vi "DemoSubClass2_SetModifiedAttributes.vi"(0 "reference in":refnum<class "DemoSubClass2.lvclass">, 2 "Attributes":T1 {"Base class"."Attribute1" format="%.2f"}, 3 "Only unlock data? (F)":bool, 4 "Unlock data if error? (T)":bool=TRUE, 5 "error in (no error)":errorcluster, 7 "Update data even if error? (F)":bool) -> (14 "reference out":refnum<class "DemoSubClass2.lvclass">, 19 "error out":errorcluster)   [LabVIEW 2020, in "DemoSubClass2.lvclass"]
doc: "This VI overwrites the attributes associated with the object reference and unlocks it for write access. If error in is set, the object is unlocked but its data will not be modified.\n\nIn order to use this VI, you must first successfully lock the object's data using this class GetAttributesToModify VI."
uses:
  DemoSubClass2.lvclass
  protected/ObjectAttributes.ctl
  DemoClass1_class/protected/ObjectAttributes.ctl
  DemoSubClass2.lvclass/DemoSubClass2.ctl
  _goop3.llb/3GOOPStates.ctl
  DemoClass1_class/DemoClass1.lvclass
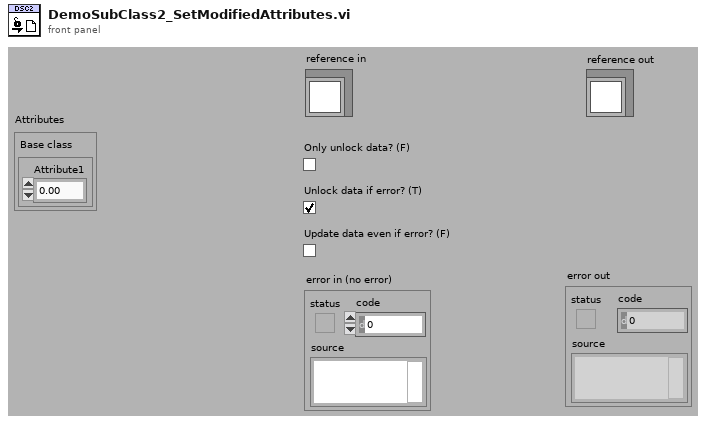
[diagram p1: front panel]
types:
  T1 = typedef "DemoSubClass2.lvclass/ObjectAttributes.ctl" = cluster{"Base class":T2}
  T2 = typedef "DemoClass1.lvclass/ObjectAttributes.ctl" = cluster{"Attribute1":dbl}
  T3 = typedef "DemoClass1.lvclass/ObjectReference.ctl" = refnum<k1>
  T4 = typedef "3GOOPStates.ctl" = enum16{"Set", "Get", "New", "Delete", "Clear", "Test and get", "Unlock data", "Information", "Look up existing", "New or look up existing", "Test and get shared", "Get shared", "Set shared", "Unlock shared", "Find dynamic method", "Register dynamic method", "Preload dynamic method", "Probe", "Cast to more generic", "Cast to more specific"}
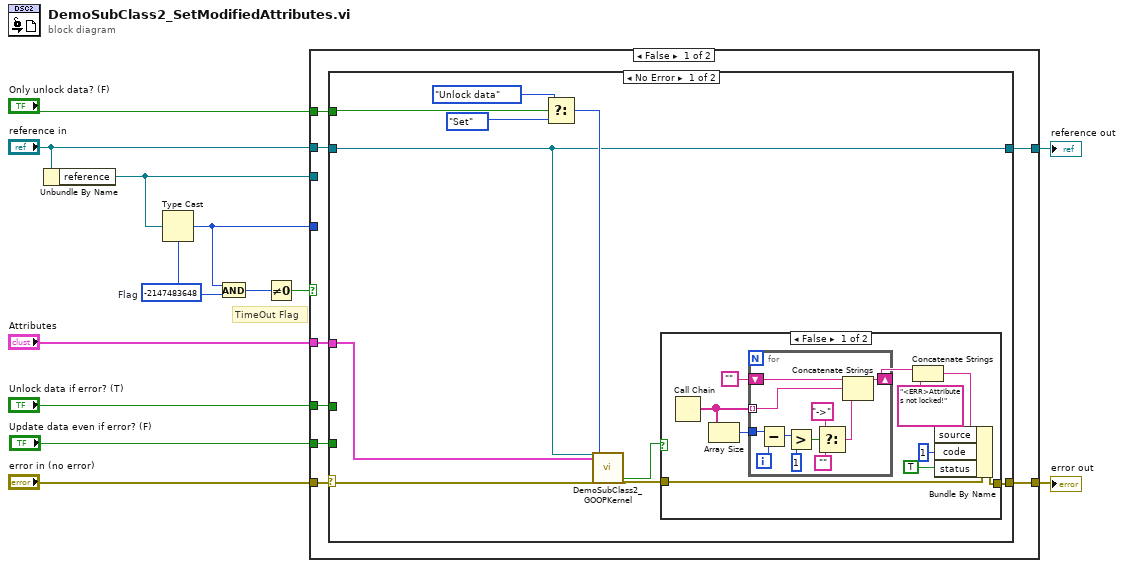
[diagram p0: block diagram]
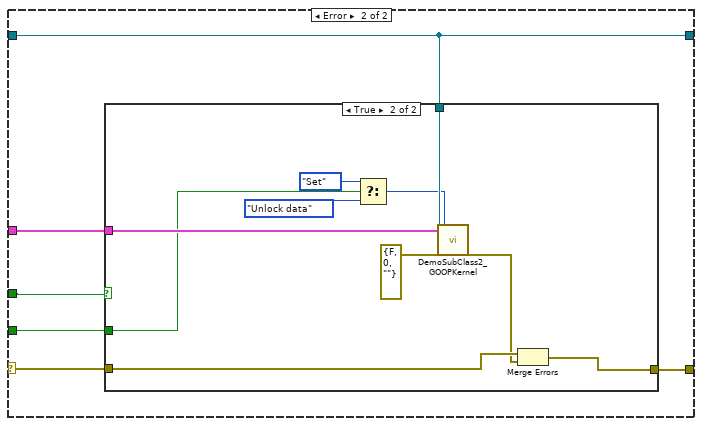
[diagram p3: hidden frame]
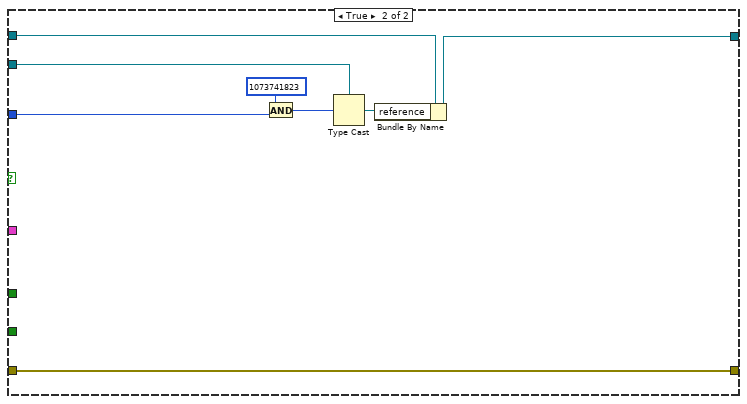
[diagram p5: hidden frame]
diagram:
  w2 = -2147483648  # Flag
  # "TimeOut Flag"
  n1 = Unbundle By Name("reference in") -> ("reference"=w5:T3)
  n2 = Type Cast(type=w2, x=w5) -> (*(type *) &x=w3:i32)
  n3 = And(x=w3, y=w2) -> (x .and. y?=w7:i32)
  n4 = Not Equal To 0?(x=w7) -> (x != 0?=w6:bool)
  n5 = case shown="False" w6 {
    tunnel: "Unlock data if error? (T)" -> [w21 _]
    tunnel: "error in (no error)" -> [w20 w71]
    tunnel: "Attributes" -> [w19 _]
    tunnel: "Only unlock data? (F)" -> [w18 _]
    tunnel: [w17 w74] -> w9
    tunnel: [w16 w71] -> w8
    tunnel: "reference in" -> [w15 w75]
    tunnel: w5 -> [_ w73]
    tunnel: w3 -> [_ w72]
    tunnel: "Update data even if error? (F)" -> [w14 _]
    frame False {
      n6 = case shown="No Error" w20 {
        selector: w20 -> [w30 w57]
        tunnel: [w22 w55] -> w17
        tunnel: w19 -> [w26 w59]
        tunnel: [w25 w56] -> w16
        tunnel: w15 -> [w22 w55]
        tunnel: w18 -> [w31 _]
        tunnel: w21 -> [_ w58]
        tunnel: w14 -> [_ w54]
        frame No Error {
          n7 = Select(t=3GOOPStates."Unlock data" ("Action"), s=w31, f=3GOOPStates."Set" ("Action")) -> (s? t:f=w27:T4)
          n8 = call "DemoSubClass2_GOOPKernel.vi"("Ref in"=w22, "Data in"=w26, "error in (no error)"=w30, "Action"=w27) -> ("Data locked?"=w23:bool, "error out"=w24:errorcluster)  [unwired: 13 in, 9 out]
          n9 = case shown="False" w23 {
            tunnel: w24 -> [w36 w53]
            tunnel: [w37 w53] -> w25
            frame False {
              n10 = Call Chain() -> (call chain=w32:string[])
              n11 = Array Size(array=w32) -> (size(s)=w40:i32)
              n12 = for {
                shift-right: [w46] -> w39
                shift-left: "" -> [w48]
                tunnel: w32 -> [w47] mode=indexing
                tunnel: w40 -> [w52]
                i -> [w51]
                n13 = Subtract(x=w52, y=w51) -> (x-y=w50:i32)
                n14 = Greater?(x=w50, y=1) -> (0:w43:bool)
                n15 = Select(t="->", s=w43, f="") -> (s? t:f=w42:string)
                n16 = Concatenate Strings(w48, w47, w42) -> (w46:string)
              }
              n17 = Concatenate Strings(w39, "<ERR>Attributes not locked!" ("Bundle Element")) -> (w35:string)
              n18 = Bundle By Name(cluster=w36, "source"=w35, "code"=1, "status"=TRUE) -> (w37:errorcluster)
            }
            frame True {
            }
          }
        }
        frame Error {
          n19 = case shown="True" w58 {
            tunnel: w57 -> [w60 w69]
            tunnel: [w60 w70] -> w56
            tunnel: w59 -> [_ w68]
            tunnel: w55 -> [_ w65]
            tunnel: w54 -> [_ w61]
            frame False {
            }
            frame True {
              n20 = Select(t=3GOOPStates."Set", s=w61, f=3GOOPStates."Unlock data" ("Action")) -> (s? t:f=w62:T4)
              n21 = call "DemoSubClass2_GOOPKernel.vi"("Ref in"=w65, "Data in"=w68, "error in (no error)"=errorcluster {"status"=FALSE, "code"=0, "source"=""}, "Action"=w62) -> ("error out"=w66:errorcluster)  [unwired: 13 in, 10 out]
              n22 = Merge Errors(w69, w66) -> (w70:errorcluster)
            }
          }
        }
      }
    }
    frame True {
      n23 = And(x=1073741823 ("x .and. y?"), y=w72) -> (x .and. y?=w78:i32)
      n24 = Type Cast(type=w73, x=w78) -> (*(type *) &x=w77:T3)
      n25 = Bundle By Name(cluster=w75, "reference"=w77) -> (w74:refnum<class "DemoSubClass2.lvclass">)
    }
  }
  "error out" <- w8
  "reference out" <- w9
